vi "fake_tool_say_hello.vi"(11 "input string":string) -> (3 "resulting string":string)   [LabVIEW 2020, in "MCP Server tests.lvlib"]
doc: "This is a fake tool to test the MCP Server. It takes a string as input and returns a string \"<input string> says hello\"."
uses:
  MCP Server tests.lvlib
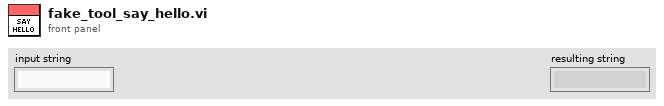
[diagram p1: front panel]
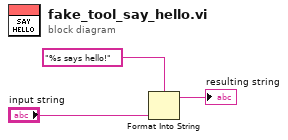
[diagram p0: block diagram]
diagram:
  n1 = Format Into String(format string="%s says hello!", "input string") -> (resulting string=→"resulting string":string)  [unwired: 2 in, 1 out]
